vi "Get Notebook Queue.vi"(2 "create if not found? (T)":bool=TRUE) -> (7 "Notebook Queue":refnum<queue>)   [LabVIEW 2021, in "Notebook.lvlib"]
uses:
  Notebook.lvlib
  Notebook Action Q Element.ctl
  Notebook Action List.ctl
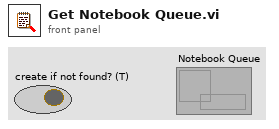
[diagram p1: front panel]
types:
  T1 = typedef "Notebook.lvlib/Notebook Action Q Element.ctl" = cluster{"Action":T2, "Variant":variant}
  T2 = typedef "Notebook.lvlib/Notebook Action List.ctl" = enum16{"Idle", "Init", "Check Content Change", "User added content", "Program added text", "Program added Picture ", "Save Notebook", "Quit", "Open", "Close", "Update Window Title"}
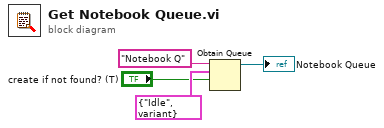
[diagram p0: block diagram]
diagram:
  n1 = Obtain Queue(name (unnamed)="Notebook Q", element data type=T1 {"Action"=enum."Idle", "Variant"=variant} ("Cluster"), create if not found? (T)="create if not found? (T)") -> (queue out=→"Notebook Queue":refnum<queue>)  [unwired: 2 in, 2 out]
